vi "Init Data.vi"(8 "error in (no error)":errorcluster, 10 "Data Object":refnum<class "Factory Plugin Framework.lvclass">=refnum, 11 "Factory Plugin Framework in":refnum<class "Factory Plugin Framework.lvclass">=refnum) -> (0 "error out":errorcluster, 3 "Factory Plugin Framework out":refnum<class "Factory Plugin Framework.lvclass">)   [LabVIEW 2018, in "Factory Plugin Framework.lvlib" / "Factory Plugin Framework.lvclass"]
uses:
  Factory Plugin Framework.lvclass
  Factory Plugin Framework.lvclass/Factory Plugin Framework.ctl
  Accessors/Write Loaded Plugins.vi
  Accessors/Write Plugin Type.vi
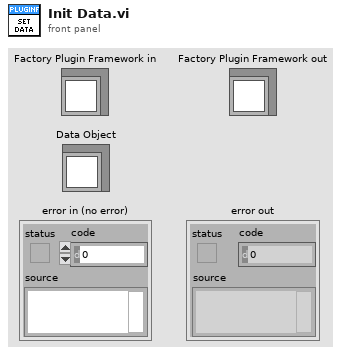
[diagram p1: front panel]
types:
  T1 = cluster{"Plugin Name":string, "Plugin Object":refnum<class>}[]
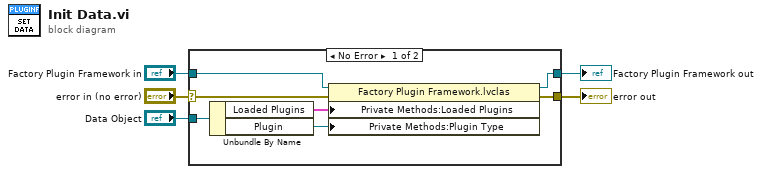
[diagram p0: block diagram]
diagram:
  n1 = case shown="No Error" "error in (no error)" {
    selector: "error in (no error)" -> [w12 w14]
    tunnel: [w11 w14] -> w4
    tunnel: "Factory Plugin Framework in" -> [w10 w13]
    tunnel: "Data Object" -> [w8 _]
    tunnel: [w9 w13] -> w1
    frame No Error {
      n2 = Unbundle By Name(w8) -> ("Loaded Plugins"=w7:T1, "Plugin"=w6:refnum<class>)
      n3 = property class="Factory Plugin Framework.lvclas"(reference=w10, error in=w12, "Private Methods:Loaded Plugins"=w7, "Private Methods:Plugin Type"=w6) -> (reference out=w9:refnum<class "Factory Plugin Framework.lvclass">, error out=w11:errorcluster)
    }
    frame Error {
    }
  }
  "error out" <- w4
  "Factory Plugin Framework out" <- w1
